vi "Takt2Winkel.vi"(11 "Taktzahl":dbl) -> (3 "Winkel (rad)":dbl)   [LabVIEW 2014]
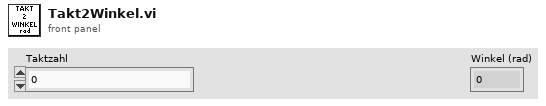
[diagram p1: front panel]
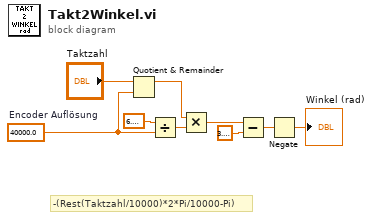
[diagram p0: block diagram]
diagram:
  w6 = 40000.0  # Encoder Auflösung
  # "-(Rest(Taktzahl/10000)*2*Pi/10000-Pi)"
  n1 = Quotient & Remainder(x="Taktzahl", y=w6) -> (x-y*floor(x/y)=w9:dbl)  [unwired: 1 out]
  n2 = Divide(x=6.283185307179586, y=w6) -> (x/y=w5:dbl)
  n3 = Multiply(x=w9, y=w5) -> (x*y=w4:dbl)
  n4 = Subtract(x=w4, y=3.141592653589793) -> (x-y=w2:dbl)
  n5 = Negate(x=w2) -> (-x=→"Winkel (rad)":dbl)
